vi "VI-Insert New VI.vi"(0 "VI in":refnum<vi>, 5 "Insert VI ref":refnum<vi>, 9 "BldArr Refnum":refnum<vi>, 11 "error in (no error)":errorcluster) -> (4 "VI out":refnum<vi>, 15 "error out":errorcluster)   [LabVIEW 2015]
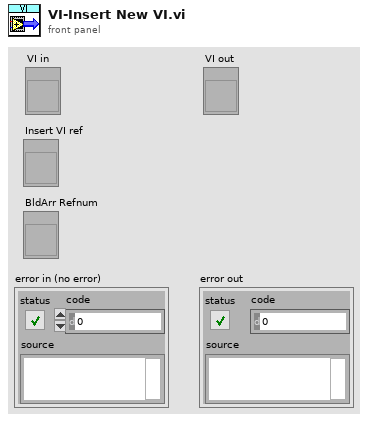
[diagram p1: front panel]
types:
  T1 = typedef "LVRectTypeDef.ctl" = cluster{"Left":i16, "Top":i16, "Right":i16, "Bottom":i16}
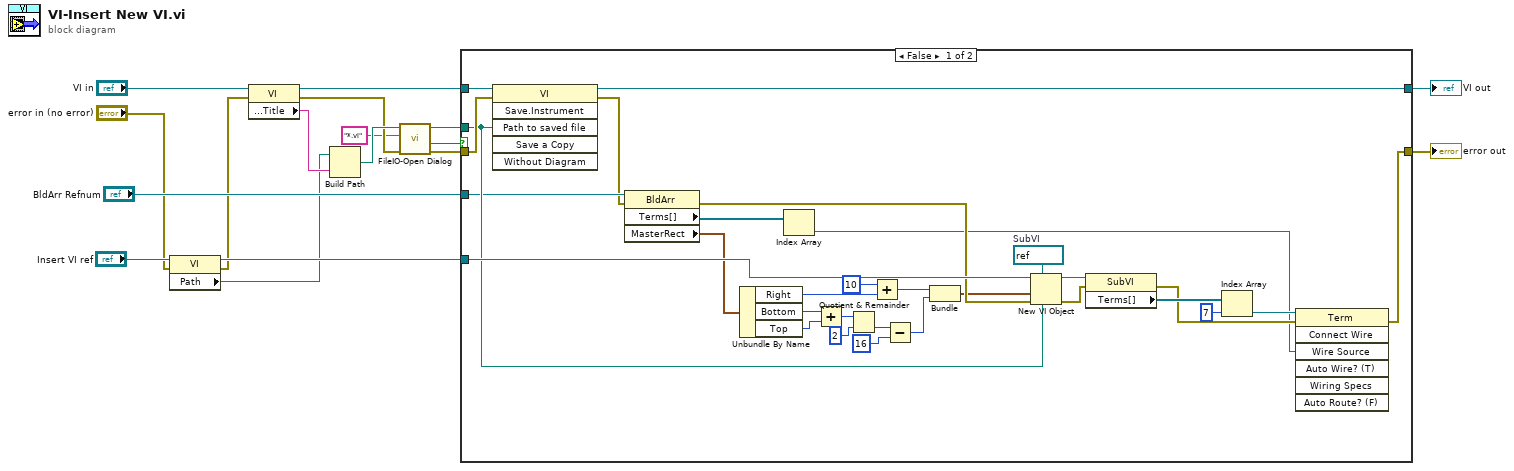
[diagram p0: block diagram]
diagram:
  n1 = property class="VI"(reference="Insert VI ref", error in="error in (no error)") -> (reference out=w4:refnum<vi>, error out=w1:errorcluster, "Path"=w3:path)
  n2 = property class="VI"(reference="VI in", error in=w1) -> (reference out=w17:refnum<vi>, error out=w13:errorcluster, "Front Panel.Title"=w16:string)
  n3 = Build Path(base path=w3, name or relative path=w16) -> (appended path=w14:path)
  n4 = call "FileIO-Open Dialog.vi"("error in"=w13, "pattern (all files)"="*.vi", "Start path"=w14) -> ("error out"=w10:errorcluster, "cancelled"=w11:bool, "selected path"=w9:path)  [unwired: 6 in]
  n5 = case shown="False" w11 {
    tunnel: w17 -> [w46 w49]
    tunnel: w4 -> [w43 _]
    tunnel: w10 -> [w45 w48]
    tunnel: w9 -> [w42 _]
    tunnel: [w44 w49] -> w8
    tunnel: [w19 w48] -> w7
    tunnel: "BldArr Refnum" -> [w41 _]
    frame False {
      w47 = refnum<vi> refnum  # SubVI
      n6 = invoke class="VI" method="Save.Instrument"(reference=w46, error in=w45, "Path to saved file"=w42) -> (reference out=w44:refnum<vi>, error out=w40:errorcluster)  [unwired: 3 in, 4 out]
      n7 = property class="BldArr"(reference=w41, error in=w40) -> (error out=w31:errorcluster, "Terms[]"=w26:refnum<vi>[], "MasterRect"=w27:T1)  [unwired: 1 out]
      n8 = Unbundle By Name(w27) -> ("Right"=w33:i16, "Bottom"=w39:i16, "Top"=w38:i16)
      n9 = Index Array(array=w26) -> (element=w18:refnum<vi>)  [unwired: 1 in]
      n10 = Add(x=w39, y=w38) -> (x+y=w37:i16)
      n11 = Quotient & Remainder(x=w37, y=i16 2) -> (floor(x/y)=w35:i16)  [unwired: 1 out]
      n12 = Add(x=i16 10, y=w33) -> (x+y=w29:i16)
      n13 = Subtract(x=w35, y=i16 16) -> (x-y=w32:i16)
      n14 = Bundle(w29, w32) -> (w30:cluster{i16, i16})  [unwired: 1 in]
      n15 = New VI Object(vi object class=w47, owner refnum=w43, position/next to=w30, 6:w42, 8:w31) -> (object refnum=w25:refnum<vi>, 0:w24:errorcluster)  [unwired: 3 in]
      n16 = property class="SubVI"(reference=w25, error in=w24) -> (error out=w20:errorcluster, "Terms[]"=w23:refnum<vi>[])  [unwired: 1 out]
      n17 = Index Array(array=w23, index=7) -> (element=w21:refnum<vi>)
      n18 = invoke class="Term" method="Connect Wire"(reference=w21, error in=w20, "Wire Source"=w18) -> (error out=w19:errorcluster)  [unwired: 4 in, 6 out]
    }
    frame True {
    }
  }
  "VI out" <- w8
  "error out" <- w7
